vi "FTW-ERR-Assert-ConditionalDisable.vi"(7 "Leave this terminal unwired.":string="Leave this terminal unwired to break the calling diagram. Nominally, this VI is only placed in a Conditional Disable Structure, intentionally breaking only platforms on which the library is not intended to run.", 11 "error in":errorcluster) -> (15 "error out":errorcluster)   [LabVIEW 2015]
doc: "Toto, I've a feeling we're not in Kansas any more.... We must be over the rainbow!"
uses:
  FTW-ERR-ThrowError.vi
  FTW-ERR-CallChain.vi
  FTW-ERR-NoErrorConstant.vi
  string/FTW-STR-ReplaceWhitespace.vi
  string/FTW-STR-Array-Delimit.vi
panel:
  # "Inputs"
  # "Outputs"
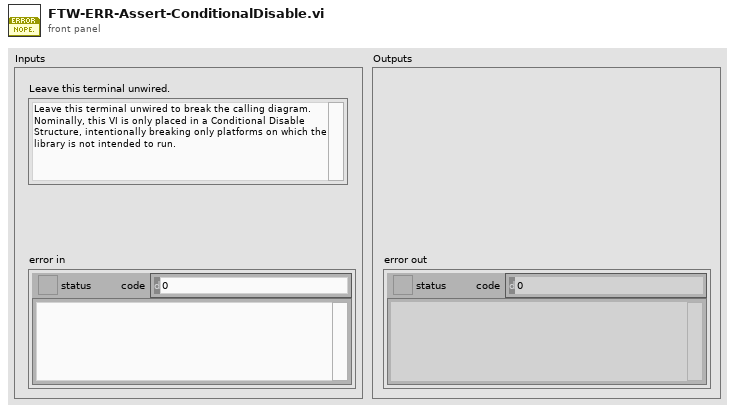
[diagram p1: front panel]
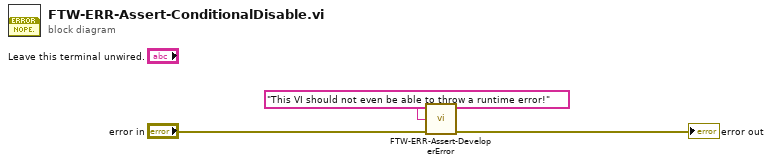
[diagram p0: block diagram]
diagram:
  n1 = call "FTW-ERR-Assert-DeveloperError.vi"("Reason this error should never happen"="This VI should not even be able to throw a runtime error!", "error in"="error in") -> ("error out"=→"error out":errorcluster)  [unwired: 13 in]
